vi "登陆后.vi"() -> ()   [LabVIEW 2019]
panel:
  in  "历史查询":bool
  in  "管理员面板":bool
  in  "停止":bool
  out "error out 3":errorcluster
  out "Data 2":string[][](array[string])
  out "最后登录时间":string
  out "error out 2":errorcluster
  out "车牌显示":T1(plugin-control)
  in  "重置":bool
  in  "开始识别":bool
  in  "请选择车牌图片":path
  out "形状定位结果":string
  out "颜色定位结果":string
  out "错误输出 2":errorcluster caption="错误输出"
  out "用户类型":string
  out "错误输出":errorcluster
  out "当前用户":string
  in  "修改密码":bool
  in  "退出登录":bool
  # "欢迎使用车牌识别系统"
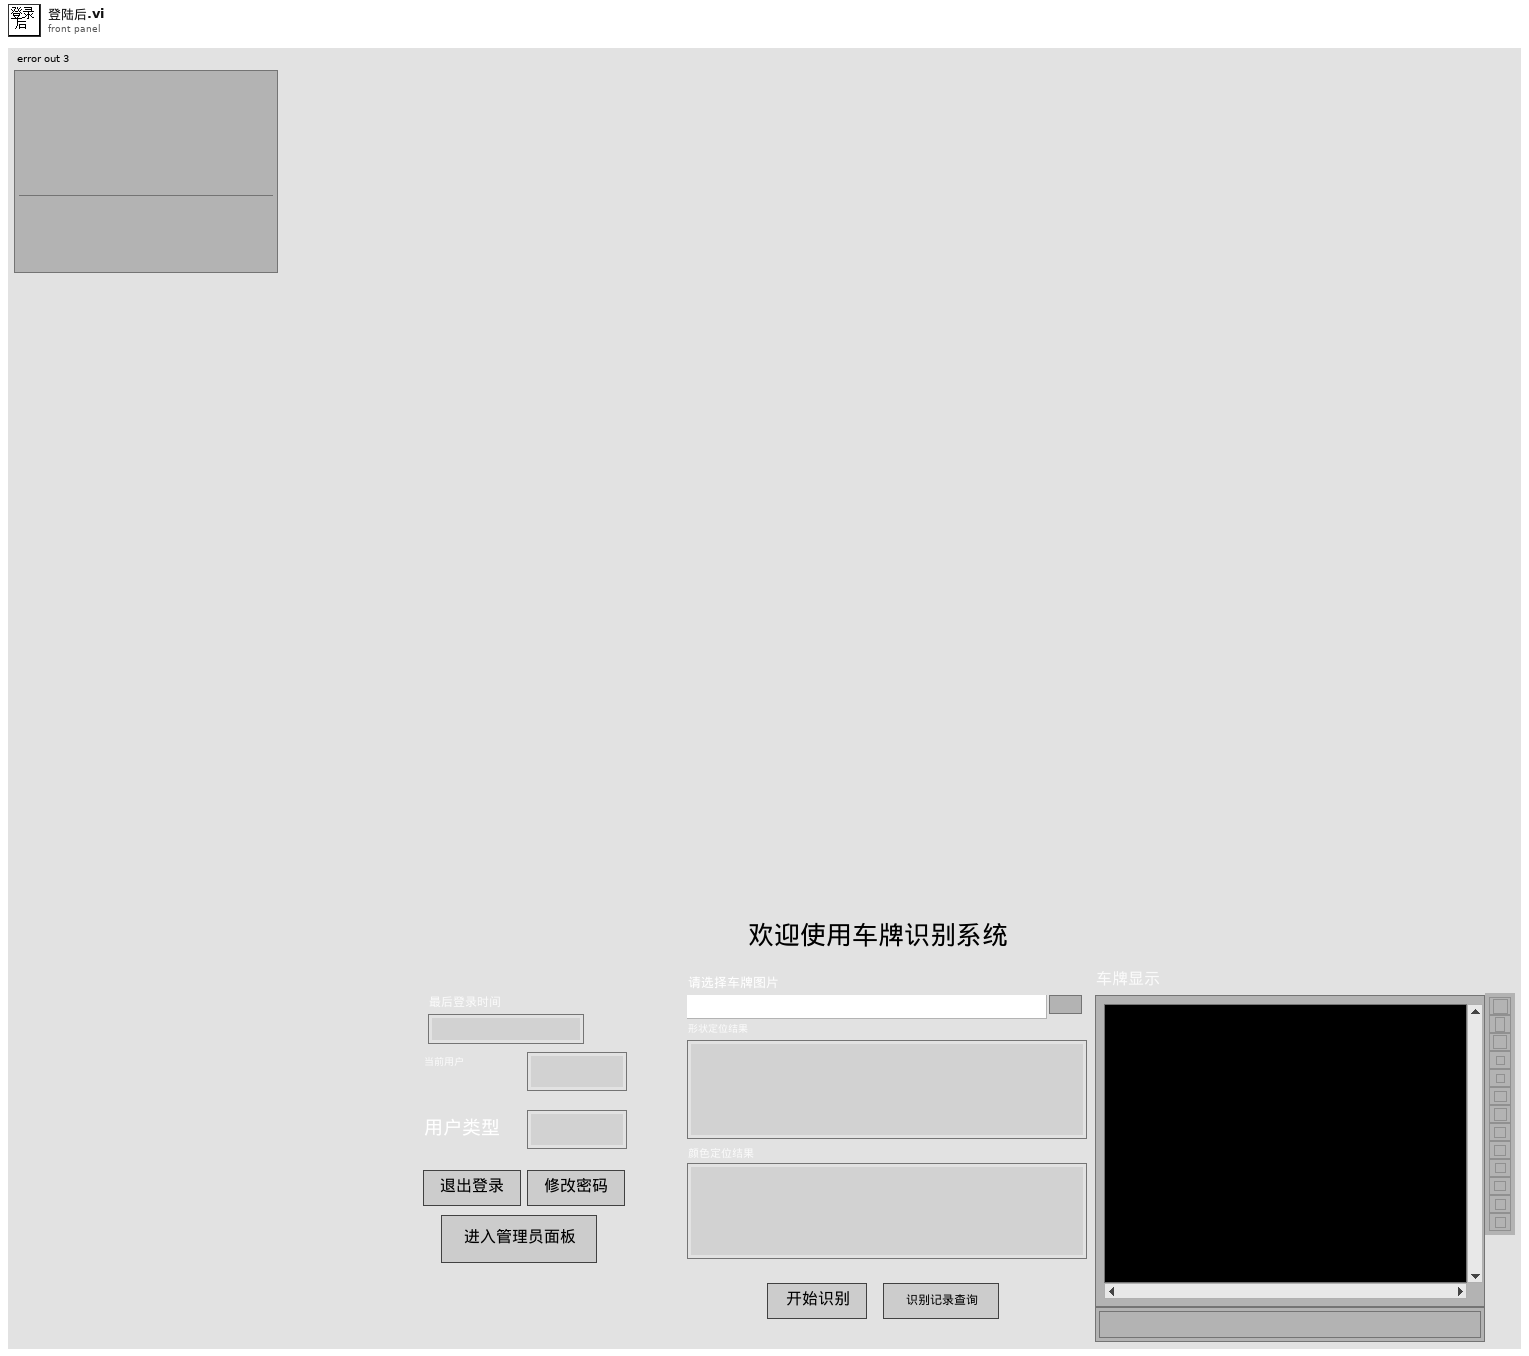
[diagram p1: front panel]
types:
  T1 = typedef "IMAQ Image.ctl" = refnum<image>
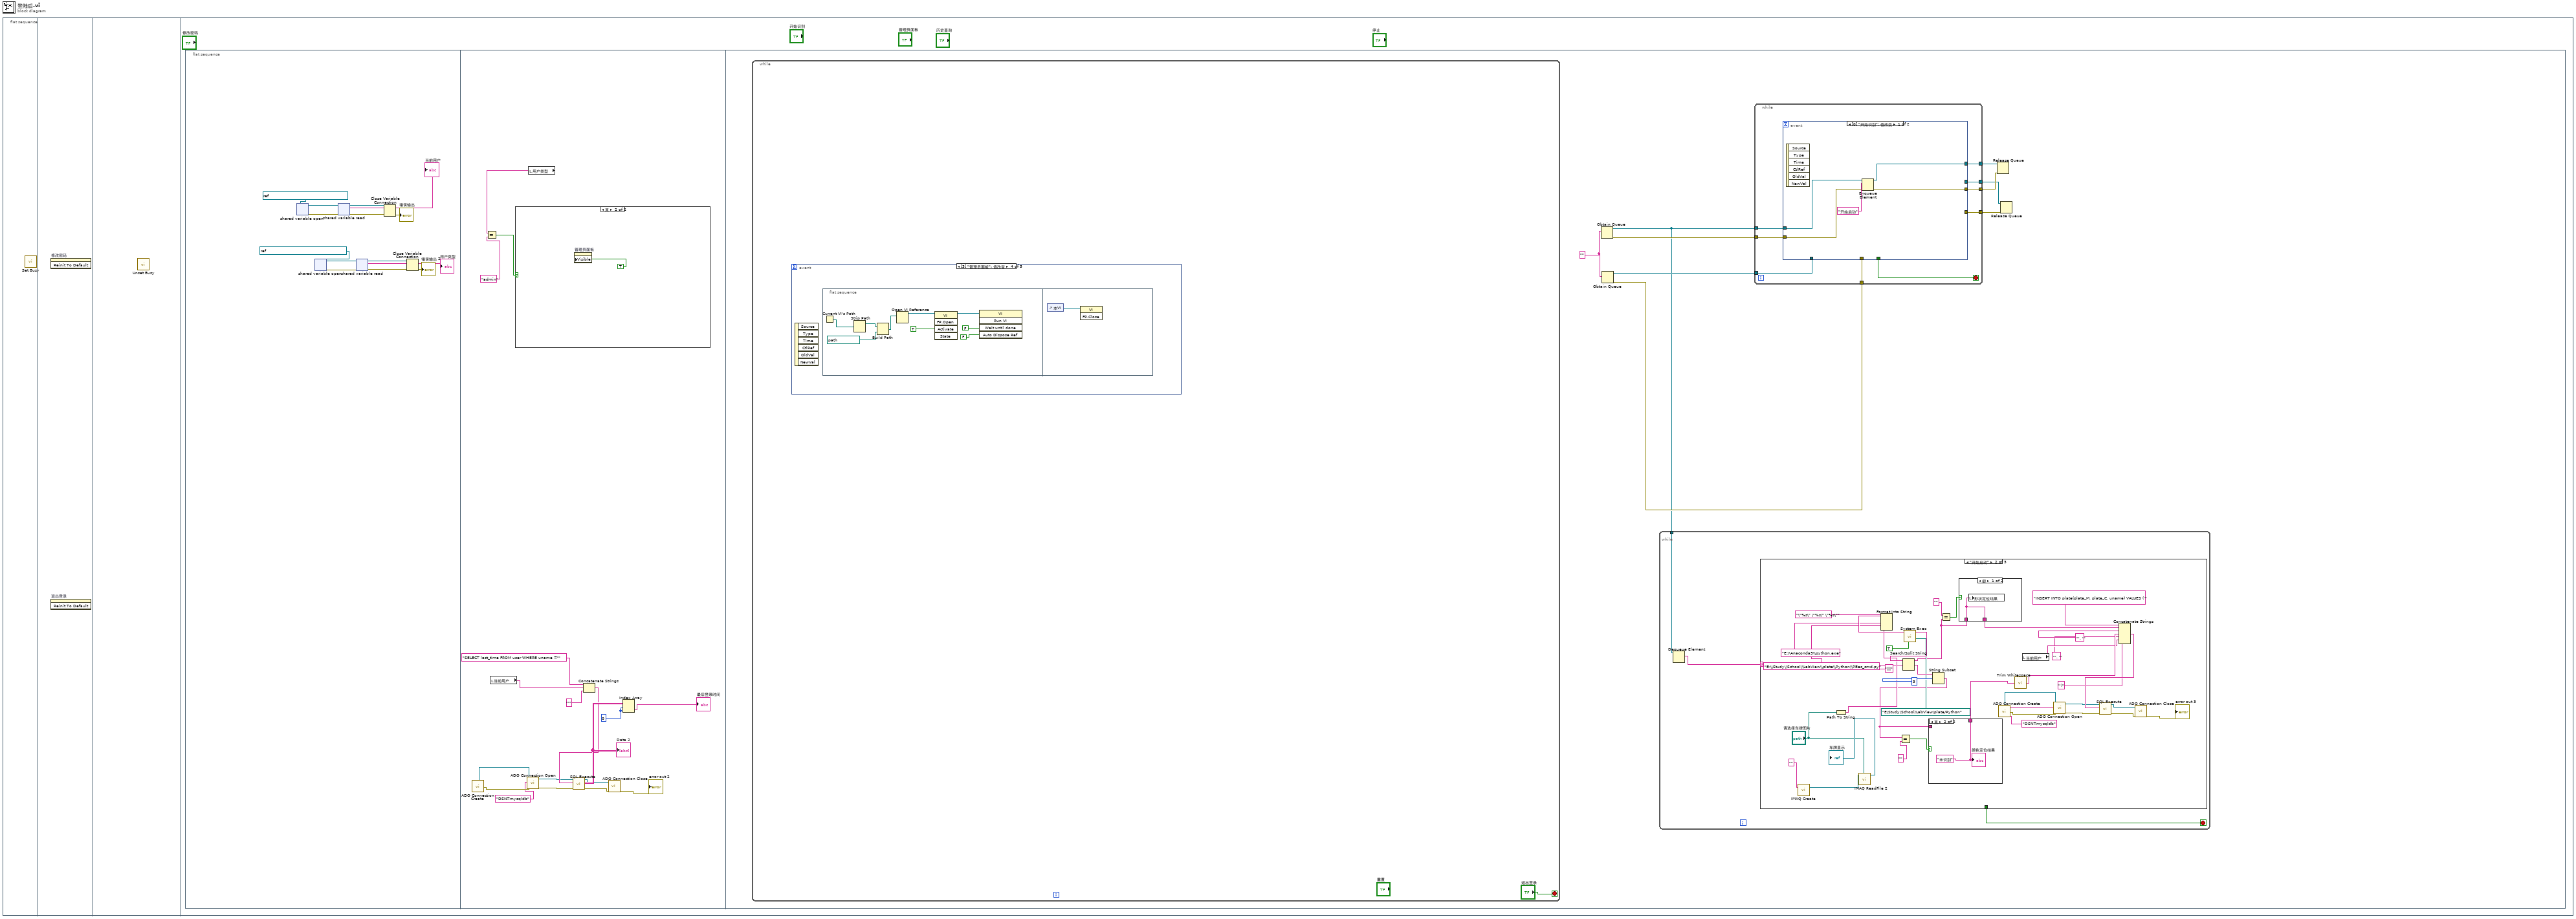
[diagram p0: block diagram]
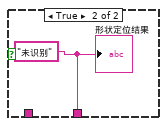
[diagram p4: hidden frame]
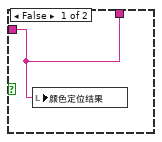
[diagram p5: hidden frame]
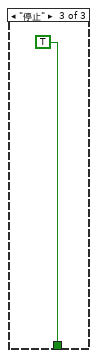
[diagram p6: hidden frame]
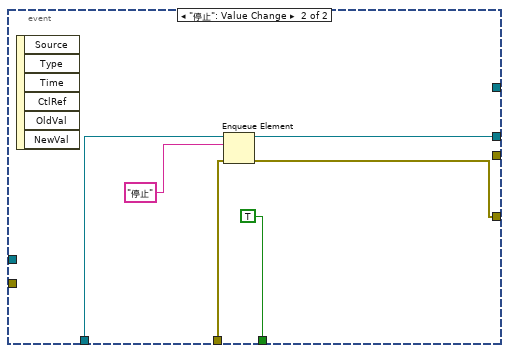
[diagram p7: hidden frame]
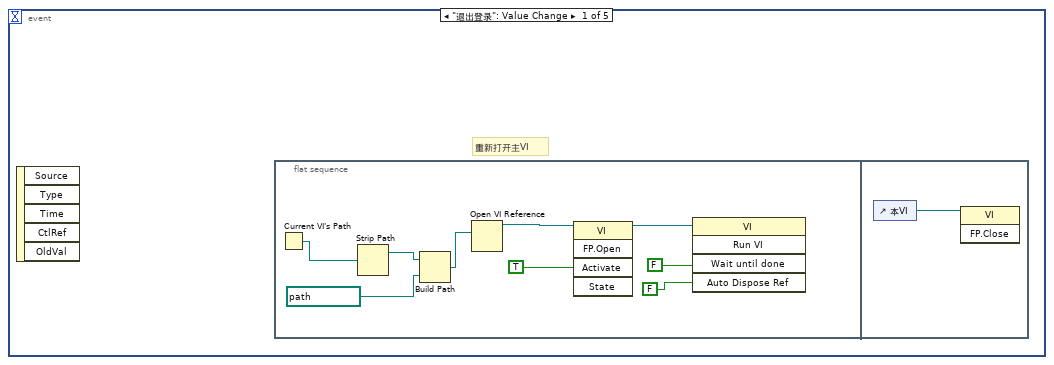
[diagram p8: hidden frame]
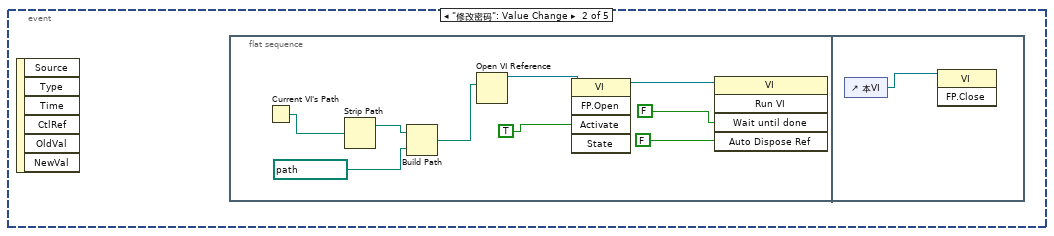
[diagram p9: hidden frame]
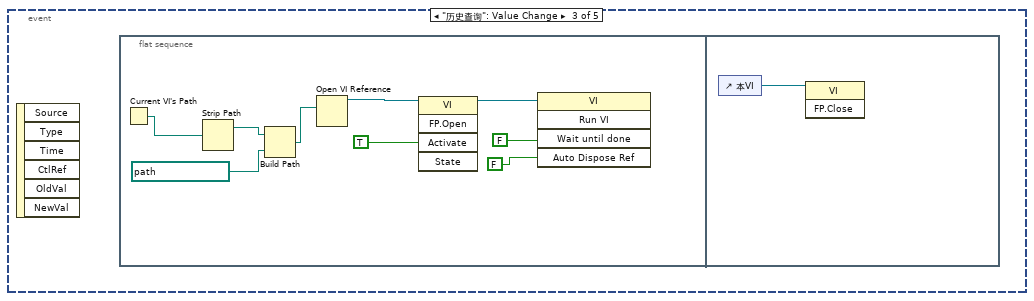
[diagram p10: hidden frame]
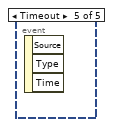
[diagram p11: hidden frame]
diagram:
  n1 = flat-sequence {
    frame #0 {
      n2 = call <vilib>:"Set Busy.vi"() -> ()  [unwired: 10 in, 2 out]
    }
    frame #1 {
      n3 = invoke on="修改密码" class="Bool" method="Reinit To Default"() -> ()  [unwired: 3 in, 3 out]
      n4 = invoke on="退出登录" class="Bool (严格)" method="Reinit To Default"() -> ()  [unwired: 3 in, 3 out]
    }
    frame #2 {
      n5 = call <vilib>:"Unset Busy.vi"() -> ()  [unwired: 11 in, 1 out]
    }
    frame #3 {
      n6 = flat-sequence {
        frame #0 {
          n7 = shared-variable-open(refnum<k21> "ni.var.psp://我的电脑/登录/登录用户" ("共享变量引用句柄输入")) -> (w3:refnum<k21>, w4:errorcluster)  [unwired: 2 in]
          n8 = shared-variable-open(refnum<k21> "ni.var.psp://localhost/登录/用户类型" ("共享变量引用句柄输入")) -> (w14:refnum<k21>, w13:errorcluster)  [unwired: 2 in]
          n9 = shared-variable-read(w3, w4) -> (w5:refnum<k21>, w6:errorcluster, →"当前用户":string)  [unwired: 1 out]
          n10 = shared-variable-read(w14, w13) -> (w12:refnum<k21>, w11:errorcluster, →"用户类型":string)  [unwired: 1 out]
          n11 = Close Variable Connection(8:w6, 11:w5) -> (0:→"错误输出":errorcluster)
          n12 = Close Variable Connection(8:w11, 11:w12) -> (0:→"错误输出 2":errorcluster)
        }
        frame #1 {
          w21 = 0
          n13 = call <userlib>:"ADO Connection Create.vi"() -> ("error out"=w23:errorcluster, "ADODB._Connection Out"=w22:refnum<k7>)  [unwired: 10 in]
          n14 = local read "当前用户"() -> (w30:string)
          n15 = call <userlib>:"ADO Connection Open.vi"("error in (no error)"=w23, "ConnectionString"="DSN=mysqldb", "ADODB._Connection In"=w22) -> ("error out"=w24:errorcluster, "ADODB._Connection Out"=w28:refnum<k7>)  [unwired: 7 in]
          n16 = local read "用户类型"() -> (w15:string)
          n17 = Equal?(x=w15, y="admin") -> (x = y?=w17:bool)
          n18 = case shown="真" w17 {
            frame False {
            }
            frame True {
              n19 = property on="管理员面板" class="Bool"("Visible"=TRUE) -> ()  [unwired: 2 in, 2 out]
            }
          }
          n20 = Concatenate Strings("SELECT last_time FROM user WHERE uname ='", w30, "'" ("字符串")) -> (w29:string)
          n21 = call <userlib>:"SQL Execute.vi"("error in (no error)"=w24, "Command Text"=w29, "ADODB._Connection In"=w28) -> ("error out"=w26:errorcluster, "Data"=w31:string[][], "ADODB._Connection Out"=w27:refnum<k7>)  [unwired: 5 in, 1 out]
          "Data 2" <- w31
          n22 = call <userlib>:"ADO Connection Close.vi"("error in (no error)"=w26, "ADODB._Connection In"=w27) -> ("error out"=→"error out 2":errorcluster)  [unwired: 8 in, 1 out]
          n23 = Index Array(array=w31, index (row)=w21, index (col)=w21) -> (element=→"最后登录时间":string)
        }
        frame #2 {
          w34 = ""
          n24 = while {
            stop <- "退出登录" stop-if-true
            n25 = event shown="[3] \"管理员面板\": 值改变" {
              selector: _ -> [_ _ _ _ _]
              dyn-events: _ -> [_ _ _ _ _]
              timeout: _ -> [_ _ _ _ _]
              event "退出登录": Value Change {
                # "重新打开主VI"
                n26 = event-data() -> ()  [unwired: 1 in, 5 out]
                n27 = flat-sequence {
                  frame #0 {
                    n28 = Current VI's Path() -> (path=w113:path)
                    n29 = Strip Path(path=w113) -> (stripped path=w112:path)  [unwired: 1 out]
                    n30 = Build Path(base path=w112, name or relative path=path "用户登录.vi") -> (appended path=w110:path)
                    n31 = Open VI Reference(vi path=w110) -> (vi reference=w115:refnum<vi>)  [unwired: 5 in, 1 out]
                    n32 = invoke class="VI" method="FP.Open"(reference=w115, "Activate"=TRUE) -> (reference out=w117:refnum<vi>)  [unwired: 3 in, 4 out]
                    n33 = invoke class="VI" method="Run VI"(reference=w117, "Wait until done"=FALSE, "Auto Dispose Ref"=FALSE) -> ()  [unwired: 2 in, 5 out]
                  }
                  frame #1 {
                    n34 = control-ref of="本VI"() -> (w119:refnum<vi>)
                    n35 = invoke class="VI" method="FP.Close"(reference=w119) -> ()  [unwired: 2 in, 3 out]
                  }
                }
              }
              event "修改密码": Value Change {
                n36 = event-data() -> ()  [unwired: 1 in, 6 out]
                n37 = flat-sequence {
                  frame #0 {
                    n38 = Current VI's Path() -> (path=w123:path)
                    n39 = Strip Path(path=w123) -> (stripped path=w122:path)  [unwired: 1 out]
                    n40 = Build Path(base path=w122, name or relative path=path "修改密码.vi") -> (appended path=w120:path)
                    n41 = Open VI Reference(vi path=w120) -> (vi reference=w124:refnum<vi>)  [unwired: 5 in, 1 out]
                    n42 = invoke class="VI" method="FP.Open"(reference=w124, "Activate"=TRUE) -> (reference out=w125:refnum<vi>)  [unwired: 3 in, 4 out]
                    n43 = invoke class="VI" method="Run VI"(reference=w125, "Wait until done"=FALSE, "Auto Dispose Ref"=FALSE) -> ()  [unwired: 2 in, 5 out]
                  }
                  frame #1 {
                    n44 = control-ref of="本VI"() -> (w129:refnum<vi>)
                    n45 = invoke class="VI" method="FP.Close"(reference=w129) -> ()  [unwired: 2 in, 3 out]
                  }
                }
              }
              event "历史查询": Value Change {
                n46 = event-data() -> ()  [unwired: 1 in, 6 out]
                n47 = flat-sequence {
                  frame #0 {
                    n48 = Current VI's Path() -> (path=w133:path)
                    n49 = Strip Path(path=w133) -> (stripped path=w132:path)  [unwired: 1 out]
                    n50 = Build Path(base path=w132, name or relative path=path "历史查询数据.vi") -> (appended path=w130:path)
                    n51 = Open VI Reference(vi path=w130) -> (vi reference=w135:refnum<vi>)  [unwired: 5 in, 1 out]
                    n52 = invoke class="VI" method="FP.Open"(reference=w135, "Activate"=TRUE) -> (reference out=w137:refnum<vi>)  [unwired: 3 in, 4 out]
                    n53 = invoke class="VI" method="Run VI"(reference=w137, "Wait until done"=FALSE, "Auto Dispose Ref"=FALSE) -> ()  [unwired: 2 in, 5 out]
                  }
                  frame #1 {
                    n54 = control-ref of="本VI"() -> (w139:refnum<vi>)
                    n55 = invoke class="VI" method="FP.Close"(reference=w139) -> ()  [unwired: 2 in, 3 out]
                  }
                }
              }
              event "管理员面板": Value Change {
                n56 = event-data() -> ()  [unwired: 1 in, 6 out]
                n57 = flat-sequence {
                  frame #0 {
                    n58 = Current VI's Path() -> (path=w143:path)
                    n59 = Strip Path(path=w143) -> (stripped path=w142:path)  [unwired: 1 out]
                    n60 = Build Path(base path=w142, name or relative path=path "管理员面板.vi") -> (appended path=w140:path)
                    n61 = Open VI Reference(vi path=w140) -> (vi reference=w145:refnum<vi>)  [unwired: 5 in, 1 out]
                    n62 = invoke class="VI" method="FP.Open"(reference=w145, "Activate"=TRUE) -> (reference out=w147:refnum<vi>)  [unwired: 3 in, 4 out]
                    n63 = invoke class="VI" method="Run VI"(reference=w147, "Wait until done"=FALSE, "Auto Dispose Ref"=FALSE) -> ()  [unwired: 2 in, 5 out]
                  }
                  frame #1 {
                    n64 = control-ref of="本VI"() -> (w149:refnum<vi>)
                    n65 = invoke class="VI" method="FP.Close"(reference=w149) -> ()  [unwired: 2 in, 3 out]
                  }
                }
              }
              event Timeout {
                n66 = event-data() -> ()  [unwired: 1 in, 3 out]
              }
            }
          }
          n67 = Obtain Queue(element data type=w34) -> (queue out=w35:refnum<queue>, error out=w41:errorcluster)  [unwired: 4 in, 1 out]
          n68 = Obtain Queue(element data type=w34) -> (queue out=w39:refnum<queue>, error out=w38:errorcluster)  [unwired: 4 in, 1 out]
          n69 = while {
            tunnel: w35 -> [w45]
            stop <- w43 stop-if-true
            n70 = Dequeue Element(queue=w45) -> (element=w44:string)  [unwired: 2 in, 3 out]
            n71 = case shown="\"开始启动\"" w44 {
              tunnel: [_ _ TRUE] -> w43
              frame "假", Default {
              }
              frame "开始启动" {
                n72 = call "IMAQ Create"("Image Name"="") -> ("New Image"=w57:T1)  [unwired: 4 in, 1 out]
                n73 = Path To String(path="请选择车牌图片") -> (string=w54:string)
                n74 = call "IMAQ ReadFile 2"("File Path"="请选择车牌图片", "Image"=w57) -> ("Image Out"=→"车牌显示":T1)  [unwired: 5 in, 4 out]
                n75 = Format Into String(format string="\"%s\" \"%s\" \"%s\"", "E:\\Anaconda3\\python.exe", "E:\\Study\\School\\LabView\\plate\\Python\\PEec_cmd.py", w54) -> (resulting string=w71:string)  [unwired: 2 in, 1 out]
                n76 = call <vilib>:"System Exec.vi"("run minimized? (F)"=TRUE, "working directory"=path "E:/Study/School/LabView/plate/Python", "command line"=w71) -> ("standard output"=w73:string)  [unwired: 5 in, 3 out]
                n77 = Search/Split String(string=w73, search string/char (-)="|||") -> (substring before match=w48:string, match + rest of string=w72:string)  [unwired: 1 in, 1 out]
                n78 = String Subset(string=w72, offset (0)=3) -> (substring=w49:string)  [unwired: 1 in]
                n79 = Equal?(x=w49, y="") -> (x = y?=w52:bool)
                n80 = case shown="真" w52 {
                  tunnel: w49 -> [w86 _]
                  tunnel: [w86 w87] -> w46
                  frame False {
                    n81 = local write "颜色定位结果"(w86) -> ()
                  }
                  frame True {
                    w87 = "未识别"
                    "颜色定位结果" <- w87
                  }
                }
                n82 = Equal?(x="", y=w48) -> (x = y?=w50:bool)
                n83 = case shown="假" w50 {
                  tunnel: w48 -> [w84 _]
                  tunnel: [w84 w85] -> w47
                  frame False {
                    n84 = local write "形状定位结果"(w84) -> ()
                  }
                  frame True {
                    w85 = "未识别"
                    "形状定位结果" <- w85
                  }
                }
                n85 = call <userlib>:"ADO Connection Create.vi"() -> ("error out"=w75:errorcluster, "ADODB._Connection Out"=w74:refnum<k7>)  [unwired: 10 in]
                n86 = call <vilib>:"Trim Whitespace.vi"("string"=w46) -> ("trimmed string"=w83:string)  [unwired: 1 in]
                n87 = local read "当前用户"() -> (w82:string)
                n88 = call <userlib>:"ADO Connection Open.vi"("error in (no error)"=w75, "ConnectionString"="DSN=mysqldb", "ADODB._Connection In"=w74) -> ("error out"=w76:errorcluster, "ADODB._Connection Out"=w80:refnum<k7>)  [unwired: 7 in]
                n89 = Concatenate Strings("INSERT INTO plate(plate_M, plate_C, uname) VALUES ('", w47, "', '" ("字符串"), w83, "', '" ("字符串"), w82, "')" ("字符串")) -> (w81:string)
                n90 = call <userlib>:"SQL Execute.vi"("error in (no error)"=w76, "Command Text"=w81, "ADODB._Connection In"=w80) -> ("error out"=w78:errorcluster, "ADODB._Connection Out"=w79:refnum<k7>)  [unwired: 5 in, 2 out]
                n91 = call <userlib>:"ADO Connection Close.vi"("error in (no error)"=w78, "ADODB._Connection In"=w79) -> ("error out"=→"error out 3":errorcluster)  [unwired: 8 in, 1 out]
              }
              frame "停止" {
              }
            }
          }
          n92 = while {
            tunnel: w35 -> [w97]
            tunnel: [w95] -> w42
            tunnel: w41 -> [w94]
            tunnel: [w93] -> w40
            tunnel: w39 -> [w92]
            tunnel: w38 -> [w91]
            tunnel: [w90] -> w37
            tunnel: [w89] -> w36
            stop <- w96 stop-if-true
            n93 = event shown="[0] \"开始识别\": 值改变" {
              selector: _ -> [_ _]
              dyn-events: _ -> [_ _]
              timeout: _ -> [_ _]
              tunnel: w97 -> [w101 _]
              tunnel: [_ TRUE] -> w96
              tunnel: [w100 _] -> w95
              tunnel: w94 -> [w99 _]
              tunnel: [w98 _] -> w93
              tunnel: w92 -> [_ w106]
              tunnel: w91 -> [_ w105]
              tunnel: [_ w104] -> w90
              tunnel: [_ w103] -> w89
              event "开始识别": Value Change {
                n94 = event-data() -> ()  [unwired: 1 in, 6 out]
                n95 = Enqueue Element(queue=w101, element="开始启动", error in (no error)=w99) -> (queue out=w100:refnum<queue>, error out=w98:errorcluster)  [unwired: 1 in, 1 out]
              }
              event "停止": Value Change {
                n96 = event-data() -> ()  [unwired: 1 in, 6 out]
                n97 = Enqueue Element(queue=w106, element="停止", error in (no error)=w105) -> (queue out=w103:refnum<queue>, error out=w104:errorcluster)  [unwired: 1 in, 1 out]
              }
            }
          }
          n98 = Release Queue(queue=w42, error in (no error)=w40) -> ()  [unwired: 1 in, 3 out]
          n99 = Release Queue(queue=w36, error in (no error)=w37) -> ()  [unwired: 1 in, 3 out]
        }
      }
    }
  }
